vi "5-20-2015.vi"() -> ()   [LabVIEW 2014]
uses:
  SPIBus0/Node/Controls/Node_Command_Sent.ctl
  <vilib>/rvi/Emulation/niFpgaGetClockAttributes.vi
  <vilib>/rvi/Emulation/niFpgaSctlEmulationGetInTimedLoop.vi
  <vilib>/rvi/Emulation/niFpgaEmulationReportErrorSimple.vi
  <vilib>/rvi/Emulation/niFpgaCriticalErrorInLSC.vi
  SPIBus0/IO Node Logic Template_SPIBus0.lvlib
panel:
  out "Received Data 3":u64
  out "Received Data 4":u64
  out "Numeric":i32
  out "Received Data 2":u64
  out "Received Data":u64
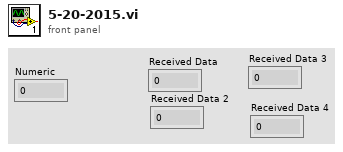
[diagram p1: front panel]
types:
  T1 = typedef "IO Node Logic Template_SPIBus0.lvlib/Node_Command_Sent.ctl" = cluster{"Device ID":u8, "Data":u64, "Command":u8, "Node ID":u8, "Misc":u8}
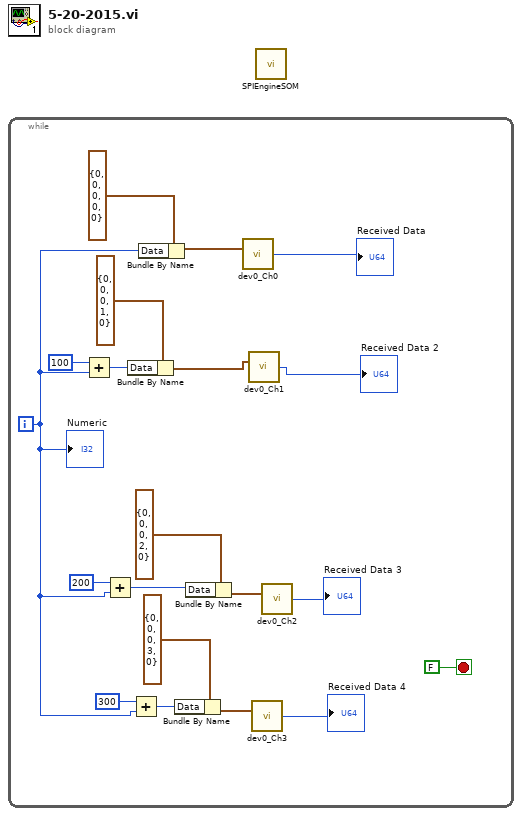
[diagram p0: block diagram]
diagram:
  n1 = while {
    i -> [w9]
    stop <- FALSE stop-if-true
    n2 = Add(x=100, y=w9) -> (x+y=w17:i32)
    n3 = Add(x=200, y=w9) -> (x+y=w10:i32)
    n4 = Bundle By Name(cluster=T1 {"Device ID"=0, "Data"=0, "Command"=0, "Node ID"=1, "Misc"=0} ("Command sent by Node"), "Data"=w17) -> (w7:T1)
    n5 = Add(x=300, y=w9) -> (x+y=w14:i32)
    n6 = Bundle By Name(cluster=T1 {"Device ID"=0, "Data"=0, "Command"=0, "Node ID"=0, "Misc"=0} ("Command sent by Node"), "Data"=w9) -> (w8:T1)
    n7 = Bundle By Name(cluster=T1 {"Device ID"=0, "Data"=0, "Command"=0, "Node ID"=3, "Misc"=0} ("Command sent by Node"), "Data"=w14) -> (w5:T1)
    n8 = Bundle By Name(cluster=T1 {"Device ID"=0, "Data"=0, "Command"=0, "Node ID"=2, "Misc"=0} ("Command sent by Node"), "Data"=w10) -> (w6:T1)
    n9 = call "dev0_Ch0.vi"("Command sent by Node"=w8) -> ("Received Data"=→"Received Data":u64)  [unwired: 14 in]
    n10 = call "dev0_Ch1.vi"("Command sent by Node"=w7) -> ("Received Data"=→"Received Data 2":u64)  [unwired: 14 in]
    n11 = call "dev0_Ch3.vi"("Command sent by Node"=w5) -> ("Received Data"=→"Received Data 4":u64)  [unwired: 14 in]
    n12 = call "dev0_Ch2.vi"("Command sent by Node"=w6) -> ("Received Data"=→"Received Data 3":u64)  [unwired: 14 in]
    "Numeric" <- w9
  }
  n13 = call "SPIEngineSOM.vi"() -> ()  [unwired: 12 in]
